vi "Mode imager in sequence.vi"(8 "error in (no error)":errorcluster) -> (0 "error out":errorcluster)   [LabVIEW 2020]
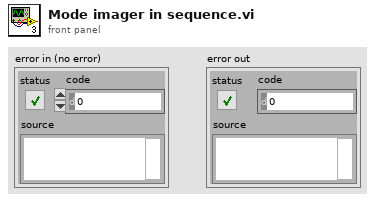
[diagram p1: front panel]
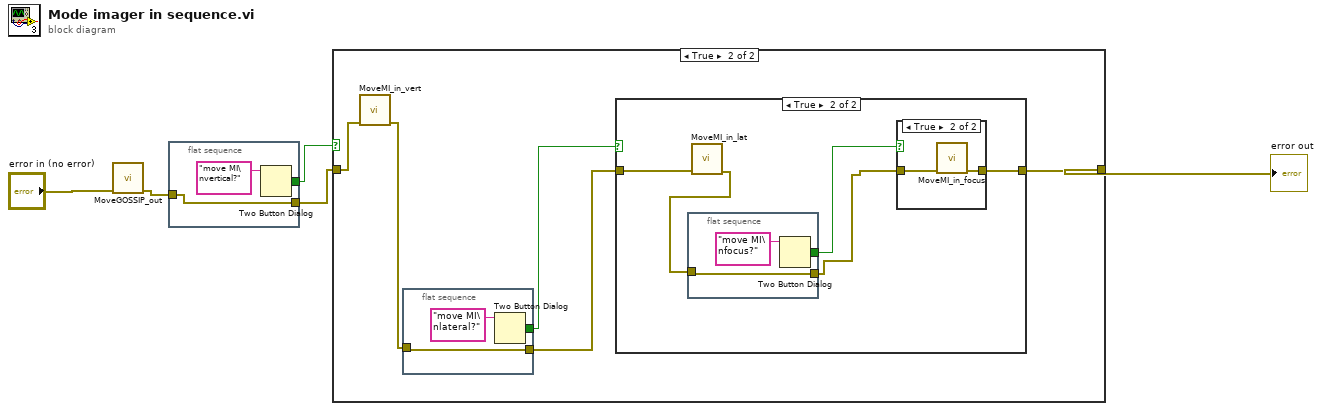
[diagram p0: block diagram]
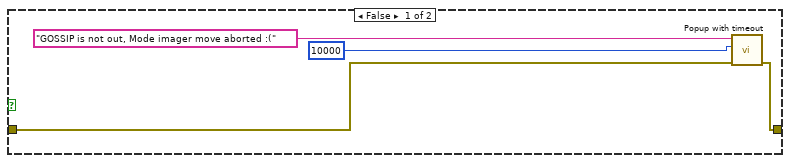
[diagram p2: hidden frame]
diagram:
  n1 = call "MoveGOSSIP_out.vi"("error in (no error)"="error in (no error)") -> ("error out"=w1:errorcluster)  [unwired: 9 in, 1 out]
  n2 = flat-sequence {
    tunnel: w1 -> [w6]
    tunnel: [w7] -> w2
    tunnel: [w6] -> w3
    frame #0 {
      n3 = Two Button Dialog(message="move MI\nvertical?") -> (T button?=w7:bool)  [unwired: 2 in]
    }
  }
  n4 = case shown="True" w2 {
    tunnel: w3 -> [w9 w14]
    tunnel: [w10 w17] -> w4
    frame False {
      n5 = call "Popup with timeout.vi"("error"=w9, "timeout"=u32 10000, "message"="GOSSIP is not out, Mode imager move aborted :(") -> ("error out"=w10:errorcluster)  [unwired: 8 in]
    }
    frame True {
      n6 = call "MoveMI_in_vert.vi"("error in (no error)"=w14) -> ("error out"=w13:errorcluster)  [unwired: 9 in, 1 out]
      n7 = flat-sequence {
        tunnel: [w31] -> w15
        tunnel: [w30] -> w16
        tunnel: w13 -> [w30]
        frame #0 {
          n8 = Two Button Dialog(message="move MI\nlateral?") -> (T button?=w31:bool)  [unwired: 2 in]
        }
      }
      n9 = case shown="True" w15 {
        tunnel: w16 -> [w18 w19]
        tunnel: [w18 w23] -> w17
        frame False {
        }
        frame True {
          n10 = flat-sequence {
            tunnel: [w25] -> w20
            tunnel: [w24] -> w21
            tunnel: w22 -> [w24]
            frame #0 {
              n11 = Two Button Dialog(message="move MI\nfocus?") -> (T button?=w25:bool)  [unwired: 2 in]
            }
          }
          n12 = call "MoveMI_in_lat.vi"("error in (no error)"=w19) -> ("error out"=w22:errorcluster)  [unwired: 9 in, 1 out]
          n13 = case shown="True" w20 {
            tunnel: w21 -> [w27 w29]
            tunnel: [w27 w28] -> w23
            frame False {
            }
            frame True {
              n14 = call "MoveMI_in_focus.vi"("error in (no error)"=w29) -> ("error out"=w28:errorcluster)  [unwired: 10 in]
            }
          }
        }
      }
    }
  }
  "error out" <- w4
